vi "add tag to default data table.vi"(8 "error in":errorcluster, 10 "system tag":refnum<class "data bus tag description.lvclass">, 11 "data dictionary in":refnum<class "data bus dictionary.lvclass">) -> (0 "error out":errorcluster, 2 "new index":i32, 3 "data dictionary out":refnum<class "data bus dictionary.lvclass">)   [LabVIEW 2013, in "data bus dictionary.lvclass"]
doc: "Adds a single tag to the default data table, converting the contained default value into a new element of the specified type, and appending that to the table."
uses:
  data bus dictionary.lvclass
  tag/data bus tag description.lvclass
  data bus dictionary.lvclass/data bus dictionary.ctl
  tag/data bus tag description.lvclass/data bus tag description.ctl
  tag/read data type.vi
  tag/read default value.vi
  tag/read raw default value.vi
  tag/default value polymorphs/read default value Double.vi
  tag/default value polymorphs/read default value I64.vi
  tag/default value polymorphs/read default value Boolean.vi
  tag/default value polymorphs/read default value Array of Double.vi
  tag/default value polymorphs/read default value Array of I64.vi
  table/data bus values.lvlib
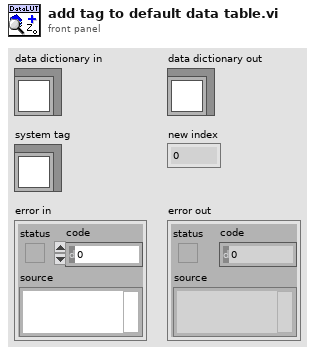
[diagram p1: front panel]
types:
  T1 = typedef "data bus values.lvlib/data table.ctl" = cluster{"Double":dbl[], "I64":i64[], "Boolean":bool[], "Array of Double":cluster{"DBL Array":dbl[]}[], "Array of I64":cluster{"I64 Array":i64[]}[], "Variant":variant[]}
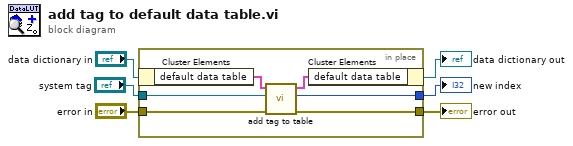
[diagram p0: block diagram]
diagram:
  n1 = in-place {
    in-place-border: "system tag" -> [w11]
    in-place-border: "error in" -> [w9]
    in-place-border: [w8] -> w2
    in-place-border: [w7] -> w1
    n2 = in-place-cluster #1("data dictionary in") -> ("default data table"=w12:T1)
    n3 = call "add tag to table.vi"("error in"=w9, "system tag"=w11, "data table in"=w12) -> ("error out"=w8:errorcluster, "new index"=w7:i32, "data table out"=w10:T1)  [unwired: 6 in]
    n4 = in-place-cluster #1("default data table"=w10) -> (→"data dictionary out":refnum<class "data bus dictionary.lvclass">)
  }
  "error out" <- w2
  "new index" <- w1
